vi "Run.vi"() -> ()   [LabVIEW 2013]
uses:
  <userlib>/_FPGA Interface Advanced Tools/FPGA Interface Base/FPGA Interface Base.lvclass
  <userlib>/KNR OS 3.0 LabVIEW Toolkit/Type Definition/Resource.ctl
  <userlib>/KNR OS 3.0 LabVIEW Toolkit/Type Definition/KNR3 Reference.ctl
panel:
  out "最終堆疊版 2":bool[][](array[boolean])
  out "Y":i32
  in  "Error":errorcluster
  in  "KNR in":T1
  out "KNR out":T1
  out "error out 4":errorcluster caption="error out"
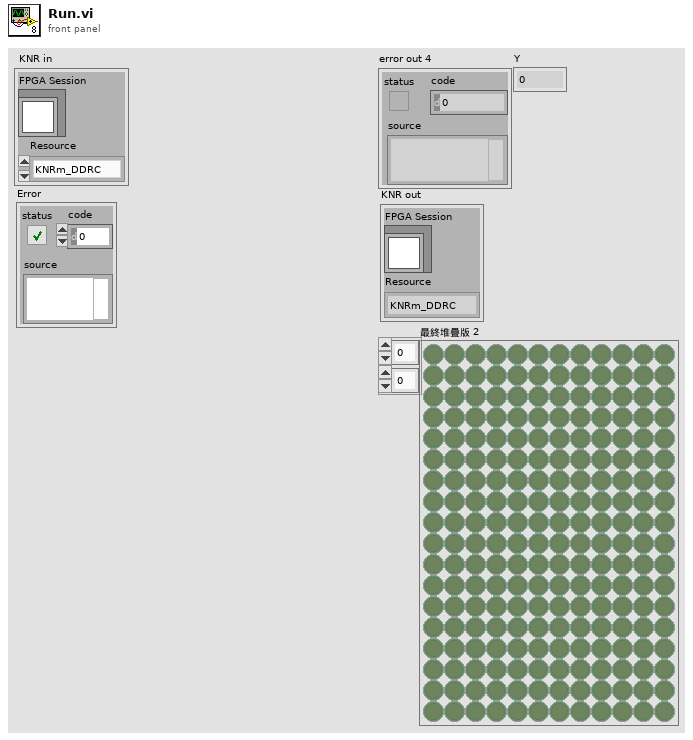
[diagram p1: front panel]
types:
  T1 = typedef "KNR3 Reference.ctl" = cluster{"FPGA Session":refnum<class "FPGA Interface Base.lvclass">, "Resource":T2}
  T2 = typedef "Resource.ctl" = enum16{"KNRm_DDRC", "KNRm_DDDD", "KNRm_DDDR", "KNRm_DDDC", "KNR"}
  T3 = cluster{"Position":cluster{"X":sgl, "Y":sgl}, "Radius":dbl, "Score":dbl}[]
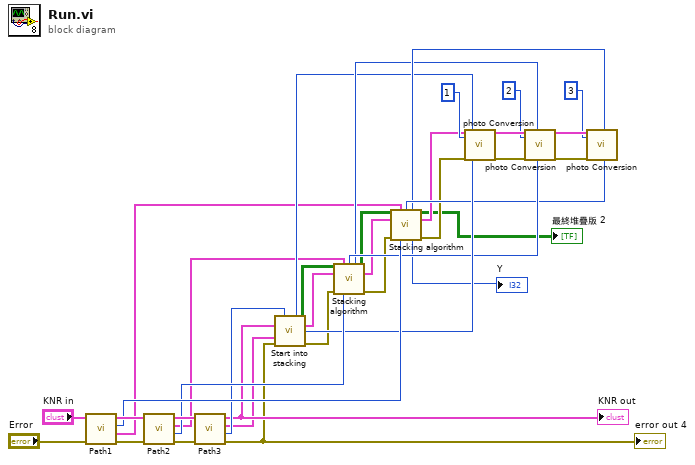
[diagram p0: block diagram]
diagram:
  n1 = call "Path1.vi"("Error"="Error", "KNR in"="KNR in") -> ("error out 4"=w36:errorcluster, "Circles (Shape Detection 1)"=w5:T3, "Number of Matches (Shape Detection 1)"=w29:i32, "KNR out"=w37:T1)  [unwired: 6 in]
  n2 = call "Path2.vi"("error in (no error)"=w36, "KNR in"=w37) -> ("error out 4"=w34:errorcluster, "Number of Matches (Shape Detection 1)"=w28:i32, "Circles (Shape Detection 1)"=w6:T3, "KNR out"=w35:T1)  [unwired: 5 in, 1 out]
  n3 = call "Path3.vi"("error in (no error)"=w34, "KNR in"=w35) -> ("error out 4"=w8:errorcluster, "Number of Matches (Shape Detection 1)"=w27:i32, "Circles (Shape Detection 1)"=w7:T3, "KNR out"=w17:T1)  [unwired: 5 in, 1 out]
  "error out 4" <- w8
  "KNR out" <- w17
  n4 = call "Start into stacking.vi"("ふ计"=w27, "KNR in"=w17, "Circles (Shape Detection 1) 2"=w7, "Error"=w8) -> ("X"=w18:i32, "最終堆疊版"=w14:bool[][], "KNR out"=w16:T1, "底盤T數"=w26:i32, "error out"=w12:errorcluster)  [unwired: 2 in, 5 out]
  n5 = call "Stacking algorithm.vi"("初始進入"=w14, "Circles (Shape Detection 1) 2"=w6, "KNR in"=w16, "Error"=w12, "ふ计"=w28) -> ("底盤T數"=w25:i32, "X"=w19:i32, "最終堆疊版 2"=w13:bool[][], "KNR out"=w15:T1, "error out"=w11:errorcluster)  [unwired: 1 in, 5 out]
  n6 = call "Stacking algorithm.vi"("初始進入"=w13, "Circles (Shape Detection 1) 2"=w5, "KNR in"=w15, "Error"=w11, "ふ计"=w29) -> ("底盤T數"=w24:i32, "X"=w20:i32, "最終堆疊版 2"=→"最終堆疊版 2":bool[][], "KNR out"=w9:T1, "Y"=→"Y":i32, "error out"=w10:errorcluster)  [unwired: 1 in, 4 out]
  n7 = call "photo Conversion.vi"("KNR in"=w9, "順序"=1, "error in"=w10, "x1"=w18, "t1"=w26) -> ("KNR out"=w33:T1, "error out"=w32:errorcluster)  [unwired: 12 in, 1 out]
  n8 = call "photo Conversion.vi"("KNR in"=w33, "順序"=2, "error in"=w32, "x2"=w19, "t2"=w25) -> ("KNR out"=w31:T1, "error out"=w30:errorcluster)  [unwired: 12 in, 1 out]
  n9 = call "photo Conversion.vi"("KNR in"=w31, "順序"=3, "error in"=w30, "x3"=w20, "t3"=w24) -> ()  [unwired: 12 in, 3 out]
